vi "Construct_Optimal_Subtrack_(11-111)-1.vi"(6 "[IN] Indexes for Jumps":i32[](array[numeric]), 8 "error IN":errorcluster, 9 "[IN] Index of recon\nstructed tracks":i32, 10 "[IN] Clusters for Re\nconstructed Tracks":T1, 11 "[IN] Still connected\ntracks in group":T2) -> (0 "error OUT":errorcluster, 2 "[OUT] Clusters for Re\nconstructed Tracks":T1)   [LabVIEW 2013]
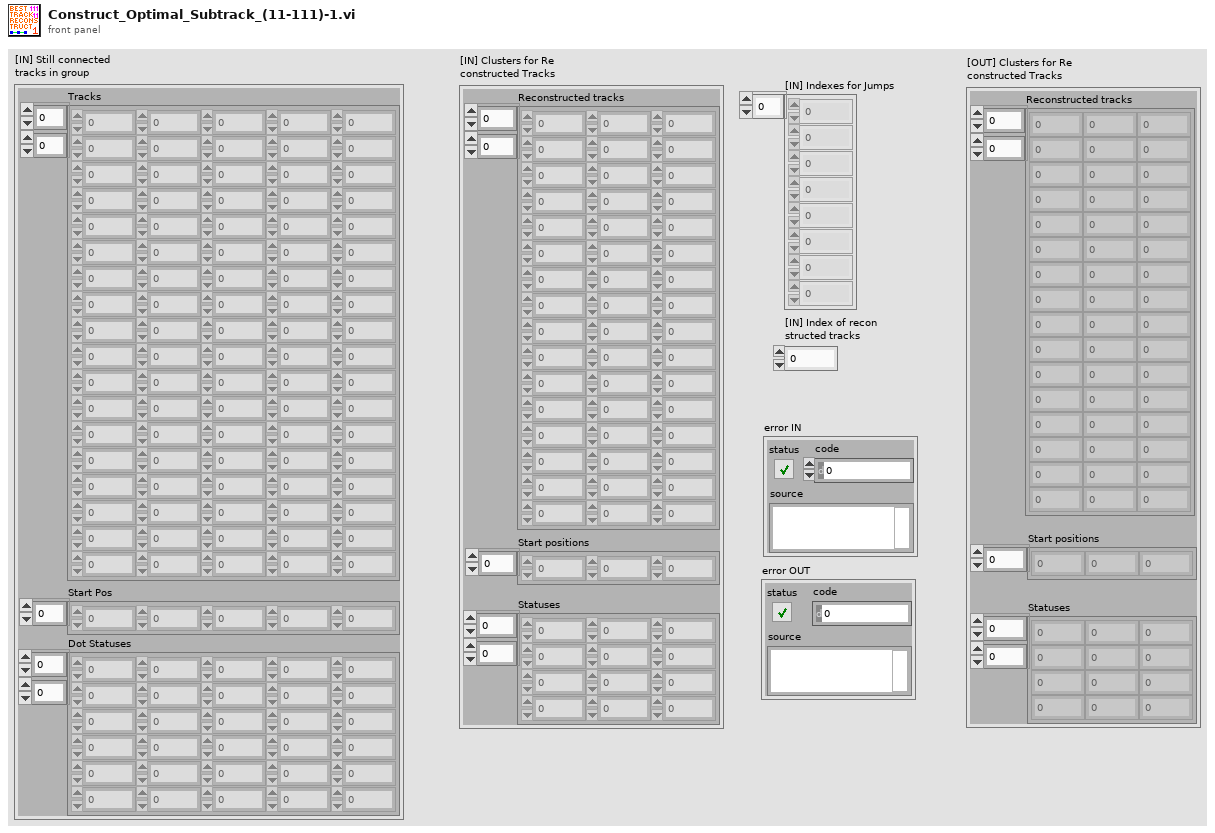
[diagram p1: front panel]
types:
  T1 = cluster{"Reconstructed tracks":dbl[][], "Start positions":i32[], "Statuses":i16[][]}
  T2 = cluster{"Tracks":dbl[][], "Start Pos":i32[], "Dot Statuses":i16[][]}
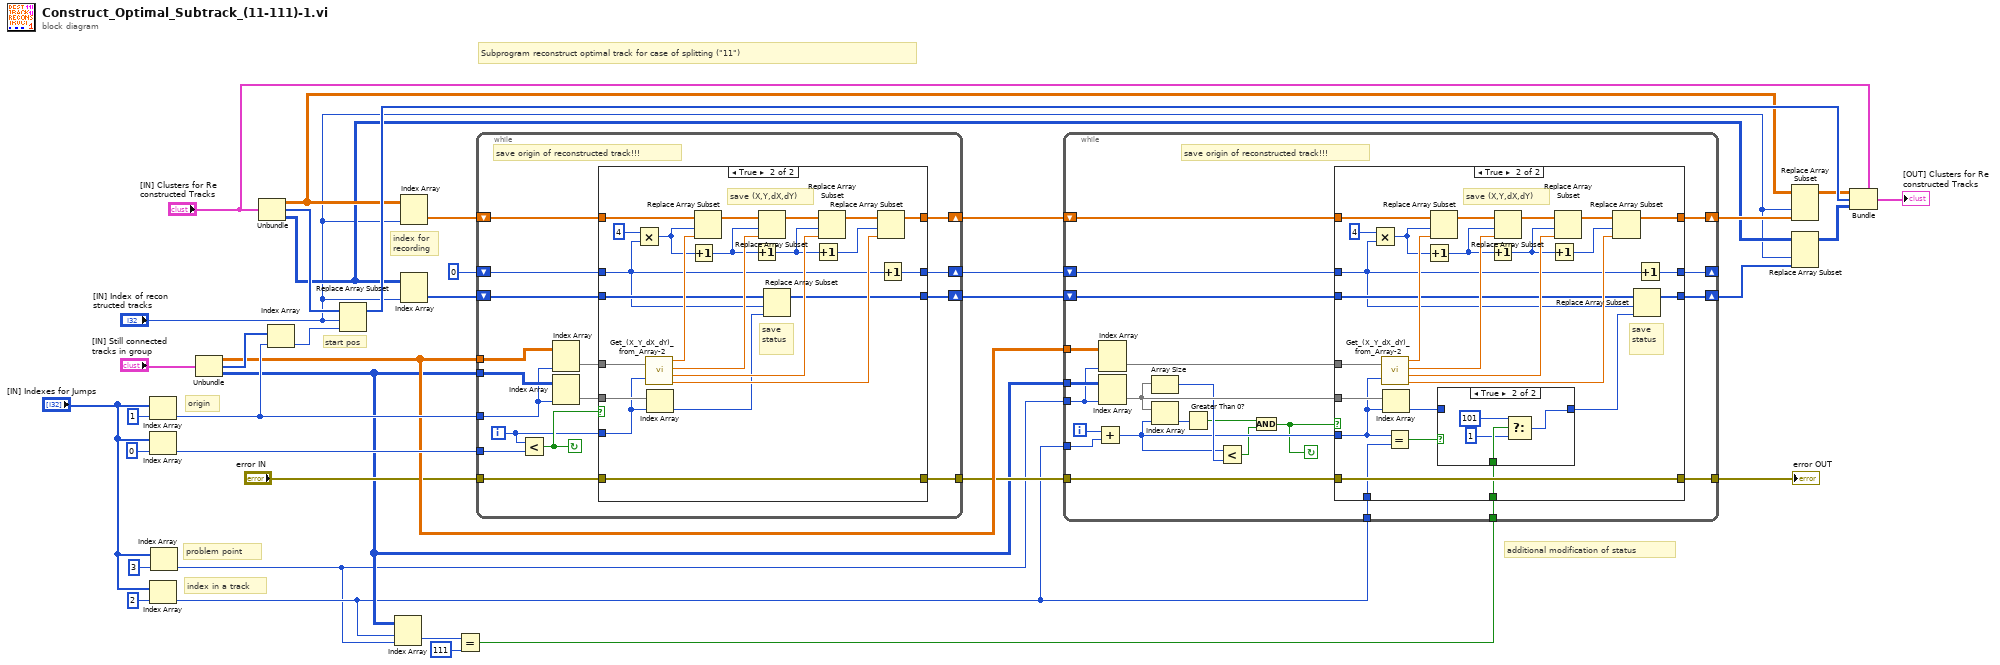
[diagram p0: block diagram]
diagram:
  # "additional modification of status"
  # "index in a track"
  # "problem point"
  # "origin"
  # "Subprogram reconstruct optimal track for case of splitting (\"11\")"
  # "index for\nrecording"
  # "start pos"
  n1 = Index Array(array="[IN] Indexes for Jumps", index=1) -> (element=w28:i32)
  n2 = Index Array(array="[IN] Indexes for Jumps", index=0) -> (element=w31:i32)
  n3 = Index Array(array="[IN] Indexes for Jumps", index=2) -> (element=w5:i32)
  n4 = Index Array(array="[IN] Indexes for Jumps", index=3) -> (element=w4:i32)
  n5 = Unbundle("[IN] Still connected\ntracks in group") -> ("Tracks"=w20:dbl[][], "Start Pos"=w29:i32[], "Dot Statuses"=w6:i16[][])
  n6 = Unbundle("[IN] Clusters for Re\nconstructed Tracks") -> ("Reconstructed tracks"=w17:dbl[][], "Start positions"=w30:i32[], "Statuses"=w14:i16[][])
  n7 = Index Array(array=w29, index=w28) -> (element=w27:i32)
  n8 = Replace Array Subset(array=w30, new element=w27, index="[IN] Index of recon\nstructed tracks") -> (w18:i32[])
  n9 = Index Array(array=w6, index (row)=w5, index (col)=w4) -> (element=w3:i16)
  n10 = Index Array(array=w17, index (col)="[IN] Index of recon\nstructed tracks") -> (element=w26:dbl[])  [unwired: 1 in]
  n11 = Index Array(array=w14, index (col)="[IN] Index of recon\nstructed tracks") -> (element=w25:i16[])  [unwired: 1 in]
  n12 = Equal?(x=w3, y=i16 111) -> (x = y?=w1:bool)
  n13 = while {
    tunnel: w31 -> [w50]
    tunnel: w20 -> [w53]
    tunnel: w6 -> [w52]
    tunnel: w28 -> [w51]
    shift-right: [w42] -> w23
    shift-left: w26 -> [w48]
    shift-right: [w40] -> w21
    shift-left: w25 -> [w44]
    shift-right: [w41] -> w22
    shift-left: 0 -> [w43]
    tunnel: "error IN" -> [w39]
    tunnel: [w38] -> w8
    i -> [w45]
    stop <- w49 continue-if-true
    # "save origin of reconstructed track!!!"
    n14 = Less?(x=w45, y=w50) -> (x < y?=w49:bool)
    n15 = Index Array(array=w53, index (col)=w51) -> (element=w47:dbl[])  [unwired: 1 in]
    n16 = Index Array(array=w52, index (col)=w51) -> (element=w46:i16[])  [unwired: 1 in]
    n17 = case shown="True" w49 {
      tunnel: w48 -> [w57 w78]
      tunnel: w47 -> [_ w80]
      tunnel: w46 -> [_ w79]
      tunnel: w45 -> [_ w63]
      tunnel: w44 -> [w55 w65]
      tunnel: [w55 w62] -> w40
      tunnel: [w57 w61] -> w42
      tunnel: w43 -> [w56 w60]
      tunnel: [w56 w59] -> w41
      tunnel: w39 -> [w54 w58]
      tunnel: [w54 w58] -> w38
      frame False {
      }
      frame True {
        # "save (X,Y,dX,dY)"
        # "save\nstatus"
        n18 = Multiply(x=4, y=w60) -> (x*y=w74:i32)
        n19 = call "Get_(X_Y_dX_dY)_from_Array-2.vi"("(X,Y,dX,dY)"=w80, "Index of Displacement"=w63) -> ("X"=w76:dbl, "Y"=w73:dbl, "dX"=w70:dbl, "dY"=w66:dbl)
        n20 = Index Array(array=w79, index=w63) -> (element=w64:i16)
        n21 = Increment(x=w74) -> (x+1=w71:i32)
        n22 = Replace Array Subset(array=w78, new element=w76, index=w74) -> (w75:dbl[])
        n23 = Increment(x=w71) -> (x+1=w69:i32)
        n24 = Replace Array Subset(array=w75, new element=w73, index=w71) -> (w72:dbl[])
        n25 = Replace Array Subset(array=w65, new element=w64, index=w60) -> (w62:i16[])
        n26 = Increment(x=w69) -> (x+1=w68:i32)
        n27 = Replace Array Subset(array=w72, new element=w70, index=w69) -> (w67:dbl[])
        n28 = Replace Array Subset(array=w67, new element=w66, index=w68) -> (w61:dbl[])
        n29 = Increment(x=w60) -> (x+1=w59:i32)
      }
    }
  }
  n30 = while {
    tunnel: w20 -> [w103]
    tunnel: w6 -> [w102]
    tunnel: w4 -> [w101]
    shift-right: [w96] -> w16
    shift-left: w23 -> [w100]
    shift-right: [w94] -> w13
    shift-left: w21 -> [w98]
    shift-right: [w95] -> _
    shift-left: w22 -> [w97]
    tunnel: w5 -> [w92]
    tunnel: w8 -> [w84]
    tunnel: [w83] -> w7
    tunnel: w5 -> [w82]
    tunnel: w1 -> [w81]
    i -> [w93]
    stop <- w85 continue-if-true
    # "save origin of reconstructed track!!!"
    n31 = Add(x=w93, y=w92) -> (x+y=w88:i32)
    n32 = Index Array(array=w103, index (col)=w101) -> (element=w99:dbl[])  [unwired: 1 in]
    n33 = Index Array(array=w102, index (col)=w101) -> (element=w91:i16[])  [unwired: 1 in]
    n34 = Array Size(array=w91) -> (size(s)=w89:i32)
    n35 = Index Array(array=w91, index=w88) -> (element=w90:i16)
    n36 = Greater Than 0?(x=w90) -> (x > 0?=w87:bool)
    n37 = Less?(x=w88, y=w89) -> (x < y?=w86:bool)
    n38 = And(x=w87, y=w86) -> (x .and. y?=w85:bool)
    n39 = case shown="True" w85 {
      tunnel: w100 -> [w107 w132]
      tunnel: w99 -> [_ w134]
      tunnel: w91 -> [_ w133]
      tunnel: w88 -> [_ w113]
      tunnel: w98 -> [w105 w119]
      tunnel: [w105 w118] -> w94
      tunnel: [w107 w117] -> w96
      tunnel: w97 -> [w106 w116]
      tunnel: [w106 w115] -> w95
      tunnel: w84 -> [w104 w114]
      tunnel: [w104 w114] -> w83
      tunnel: w82 -> [_ w112]
      tunnel: w81 -> [_ w108]
      frame False {
      }
      frame True {
        # "save (X,Y,dX,dY)"
        # "save\nstatus"
        n40 = Multiply(x=4, y=w116) -> (x*y=w128:i32)
        n41 = call "Get_(X_Y_dX_dY)_from_Array-2.vi"("(X,Y,dX,dY)"=w134, "Index of Displacement"=w113) -> ("X"=w130:dbl, "Y"=w127:dbl, "dX"=w124:dbl, "dY"=w120:dbl)
        n42 = Index Array(array=w133, index=w113) -> (element=w110:i16)
        n43 = Equal?(x=w113, y=w112) -> (x = y?=w111:bool)
        n44 = Increment(x=w128) -> (x+1=w125:i32)
        n45 = Replace Array Subset(array=w132, new element=w130, index=w128) -> (w129:dbl[])
        n46 = case shown="True" w111 {
          tunnel: w110 -> [w135 _]
          tunnel: [w135 w136] -> w109
          tunnel: w108 -> [_ w139]
          frame False {
          }
          frame True {
            n47 = Select(t=i16 101 ("element"), s=w139, f=i16 1 ("element")) -> (s? t:f=w136:i16)
          }
        }
        n48 = Increment(x=w125) -> (x+1=w123:i32)
        n49 = Replace Array Subset(array=w129, new element=w127, index=w125) -> (w126:dbl[])
        n50 = Increment(x=w123) -> (x+1=w122:i32)
        n51 = Replace Array Subset(array=w126, new element=w124, index=w123) -> (w121:dbl[])
        n52 = Replace Array Subset(array=w121, new element=w120, index=w122) -> (w117:dbl[])
        n53 = Replace Array Subset(array=w119, new element=w109, index=w116) -> (w118:i16[])
        n54 = Increment(x=w116) -> (x+1=w115:i32)
      }
    }
  }
  "error OUT" <- w7
  n55 = Replace Array Subset(array=w17, new element=w16, index (col)="[IN] Index of recon\nstructed tracks") -> (w15:dbl[][])  [unwired: 1 in]
  n56 = Replace Array Subset(array=w14, new element=w13, index (col)="[IN] Index of recon\nstructed tracks") -> (w11:i16[][])  [unwired: 1 in]
  n57 = Bundle(cluster="[IN] Clusters for Re\nconstructed Tracks", "Reconstructed tracks"=w15, "Start positions"=w18, "Statuses"=w11) -> (→"[OUT] Clusters for Re\nconstructed Tracks":T1)
